vi "Synapse Interface Test.vi"() -> ()   [LabVIEW 2015]
uses:
  sub VIs/TDT-Sys Mode Enum.ctl
  <vilib>/httpClient/LabVIEWHTTPClient.lvlib
panel:
  out "mode":T1
  out "error out":errorcluster
  in  "error in (no error)":errorcluster
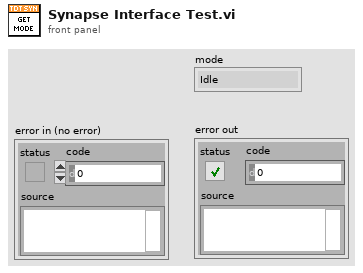
[diagram p1: front panel]
types:
  T1 = typedef "TDT-Sys Mode Enum.ctl" = enum16{"Idle", "Standby", "Preview", "Record"}
  T2 = typedef "LabVIEWHTTPClient.lvlib/ClientHandle.ctl" = refnum<k1>
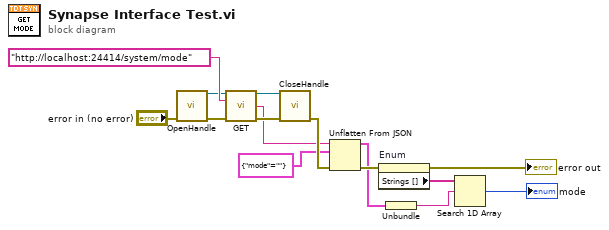
[diagram p0: block diagram]
diagram:
  n1 = call <vilib>:"OpenHandle.vi"("error in (no error)"="error in (no error)") -> ("client handle out"=w12:T2, "error out"=w11:errorcluster)  [unwired: 13 in]
  n2 = call <vilib>:"GET.vi"("client handle"=w12, "url"="http://localhost:24414/system/mode", "error in (no error)"=w11) -> ("client handle out"=w14:T2, "body"=w8:string, "error out"=w15:errorcluster)  [unwired: 9 in, 1 out]
  n3 = call <vilib>:"CloseHandle.vi"("client handle"=w14, "error in (no error)"=w15) -> ("error out"=w10:errorcluster)  [unwired: 13 in]
  n4 = Unflatten From JSON(JSON string=w8, type and defaults=cluster{"mode":string} {"mode"=""} ("Cluster"), error in (no error)=w10) -> (value=w4:cluster{"mode":string}, error out=w6:errorcluster)  [unwired: 4 in]
  n5 = property on="Enum" class="Enum (strict)"(error in=w6) -> (error out=→"error out":errorcluster, "Strings []"=w5:string[])  [unwired: 1 in, 1 out]
  n6 = Unbundle(w4) -> ("mode"=w3:string)
  n7 = Search 1D Array(1D array=w5, element=w3) -> (index of element=→"mode":i32)  [unwired: 1 in]
